vi "ConfigLoadTest.vi"() -> ()   [LabVIEW 2013, in "J1939 tests.lvlib"]
uses:
  J1939 tests.lvlib
  <vilib>/NI/DCAF/Tag Editor Core/Framework Configuration Classes/platypus configuration/targets cluster.ctl
  <vilib>/NI/DCAF/Tag Editor Core/Framework Configuration Classes/target configuration/PL_Target Configuration.lvclass
  <vilib>/NI/DCAF/Tag Editor Core/Framework Configuration Classes/platypus configuration/engines cluster.ctl
  <vilib>/NI/Module Execution Interface/Engine Configuration/engine configuration.lvclass
  <vilib>/NI/Tag Bus Module Framework/module configuration/TBM module configuration.lvclass
  module/configuration/XNET Settings.ctl
  module/configuration/Line.ctl
  <vilib>/NI/Tag Bus Module Framework/channel/TBM channel.lvclass
  module/configuration/J1939 configuration.lvclass
  module/configuration/J1939 configuration.lvclass/J1939 configuration.ctl
  module/configuration/Read XNET Settings.vi
  module/configuration/Read Lines.vi
  <vilib>/NI/Configuration Framework/tree serializer/NISE_CEF_TreeSerializer.lvlib
  <vilib>/NI/DCAF/Tag Editor Core/Framework Configuration Classes/flattened data interface/PL_Serialization Interface.lvlib
  <vilib>/NI/DCAF/Tag Editor Core/Framework Configuration Classes/platypus configuration/PLConfigurationSerializer.lvlib
panel:
  out "Customize:Properties:Lines":T1[][](array[typedef])
  out "Array":T2[](array[typedef])
  out "error out":errorcluster
  out "targets cluster out":T3
  in  "file path":path=path "c:/TestConfig.pcfg"
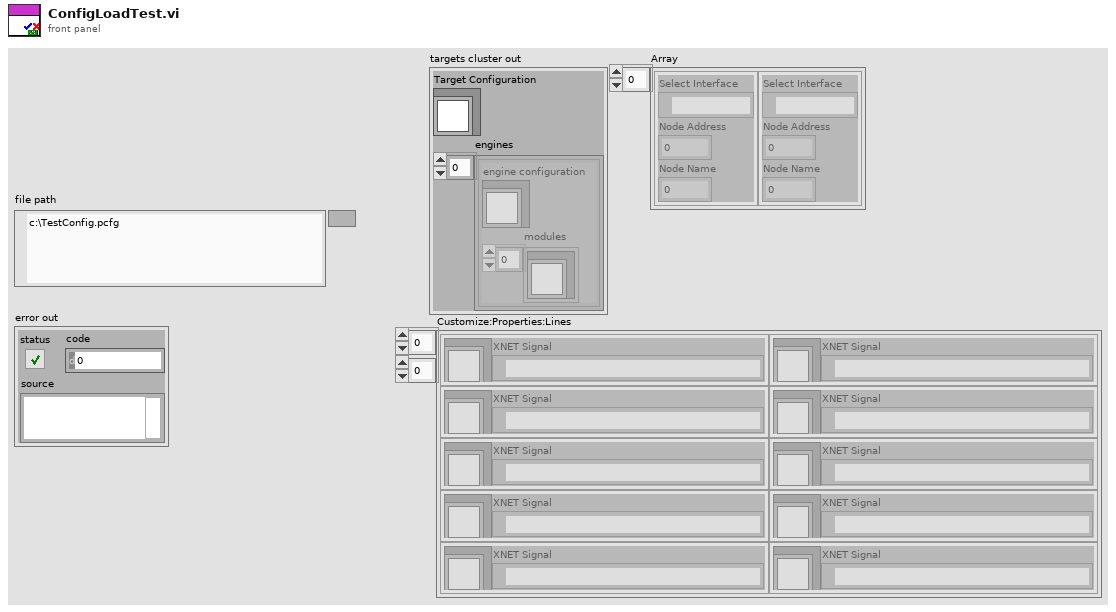
[diagram p1: front panel]
types:
  T1 = typedef "J1939 configuration.lvclass/Line.ctl" = cluster{"channel":refnum<class "TBM channel.lvclass">, "XNET Signal":refnum<k21>}
  T2 = typedef "J1939 configuration.lvclass/XNET Settings.ctl" = cluster{"Select Interface":refnum<k21>, "Node Address":u8, "Node Name":u64}
  T3 = typedef "PLConfigurationSerializer.lvlib/targets cluster.ctl" = cluster{"Target Configuration":refnum<class "PL_Target Configuration.lvclass">, "engines":T4[]}
  T4 = typedef "PLConfigurationSerializer.lvlib/engines cluster.ctl" = cluster{"engine configuration":refnum<class "engine configuration.lvclass">, "modules":refnum<class "TBM module configuration.lvclass">[]}
  T5 = typedef "NISE_CEF_TreeSerializer.lvlib/base file format.ctl" = cluster{"version":string, "data":string}
  T6 = typedef "NISE_CEF_TreeSerializer.lvlib/flat hierarchy.ctl" = cluster{"hierarchy structure":T7, "instance data":T9[]}
  T7 = typedef "NISE_CEF_TreeSerializer.lvlib/full hierarchy.ctl" = cluster{"root":string, "hierarchy":T8[]}
  T8 = typedef "NISE_CEF_TreeSerializer.lvlib/hierarchy element.ctl" = cluster{"current node":string, "children":string[]}
  T9 = typedef "NISE_CEF_TreeSerializer.lvlib/instance data.ctl" = cluster{"ID":string, "Alias":string, "class":string, "version":string, "data":string}
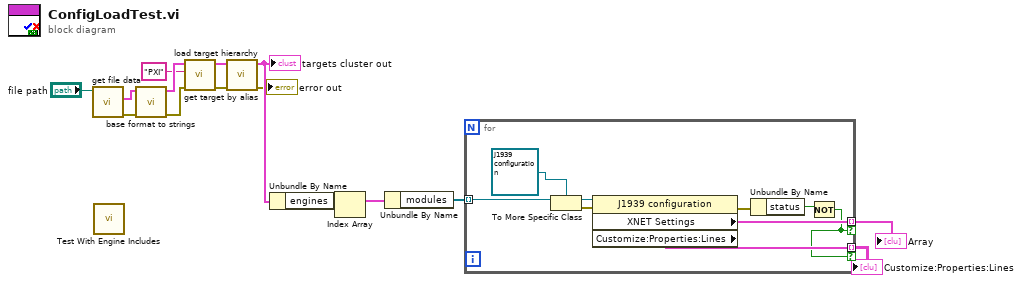
[diagram p0: block diagram]
diagram:
  n1 = call <vilib>:"get file data.vi"("Path"="file path") -> ("error out"=w14:errorcluster, "format"=w15:T5)  [unwired: 9 in]
  n2 = call "Test With Engine Includes.vi"() -> ()  [unwired: 12 in]
  n3 = call <vilib>:"base format to strings.vi"("error in"=w14, "format"=w15) -> ("error out"=w9:errorcluster, "data"=w12:T6)  [unwired: 8 in]
  n4 = call <vilib>:"get target by alias.vi"("error in"=w9, "alias"="PXI", "system hierarchy"=w12) -> ("error out"=w10:errorcluster, "target hierarchy"=w11:T6)  [unwired: 7 in]
  n5 = call <vilib>:"load target hierarchy.vi"("error in"=w10, "target hierarchy"=w11) -> ("error out"=→"error out":errorcluster, "targets cluster out"=w7:T3)  [unwired: 8 in]
  "targets cluster out" <- w7
  n6 = Unbundle By Name(w7) -> ("engines"=w6:T4[])
  n7 = Index Array(array=w6) -> (element=w1:T4)  [unwired: 1 in]
  n8 = Unbundle By Name(w1) -> ("modules"=w2:refnum<class "TBM module configuration.lvclass">[])
  n9 = for {
    tunnel: w2 -> [w24] mode=indexing
    tunnel: [w21] -> w5 mode=indexing if=w16
    tunnel: [w20] -> w4 mode=indexing if=w16
    n10 = To More Specific Class(target class=refnum<class "J1939 configuration.lvclass"> refnum ("J1939 configuration"), reference=w24) -> (specific class reference=w22:refnum<class "J1939 configuration.lvclass">, error out=w19:errorcluster)  [unwired: 1 in]
    n11 = property class="J1939 configuration"(reference=w22, error in=w19) -> (error out=w18:errorcluster, "XNET Settings"=w21:T2, "Customize:Properties:Lines"=w20:T1[])  [unwired: 1 out]
    n12 = Unbundle By Name(w18) -> ("status"=w17:bool)
    n13 = Not(x=w17) -> (.not. x?=w16:bool)
  }
  "Array" <- w5
  "Customize:Properties:Lines" <- w4
